vi "MultiGrid.vi"() -> ()   [LabVIEW 2014]
uses:
  <userlib>/Nanonis Prog Interface V5/Nanonis Prog Interface.lvlib
panel:
  in  "Cloud Grid":bool=TRUE
  in  "GridSettings":T1={"Imaging Current"=5e-11, "STS Current"=1e-09, "Start value (V)"=-0.05, "End value (V)"=0.05, "Number of points (0=no change)"=256, "File name"="single_mol_shortSTS", "DC pixel"=64.0, "Grid X"=0.0, "Grid Y"=0.0, "Sweeps"=8.0}
  in  "Polling (s)":u32=600
  out "Status":string="Waiting for grid to start"
  out "#Grids":i32=2
  out "MultiGrid":i32(listbox)
  # "0 for no change"
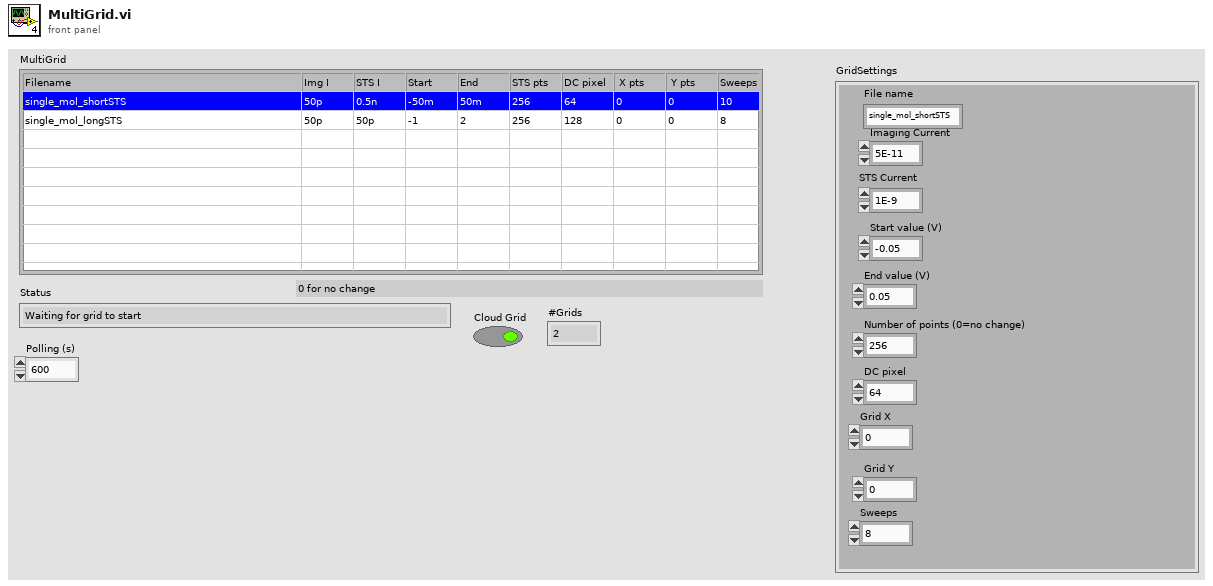
[diagram p1: front panel]
types:
  T1 = cluster{"Imaging Current":sgl, "STS Current":sgl, "Start value (V)":sgl, "End value (V)":sgl, "Number of points (0=no change)":i32, "File name":string, "DC pixel":dbl, "Grid X":dbl, "Grid Y":dbl, "Sweeps":dbl}
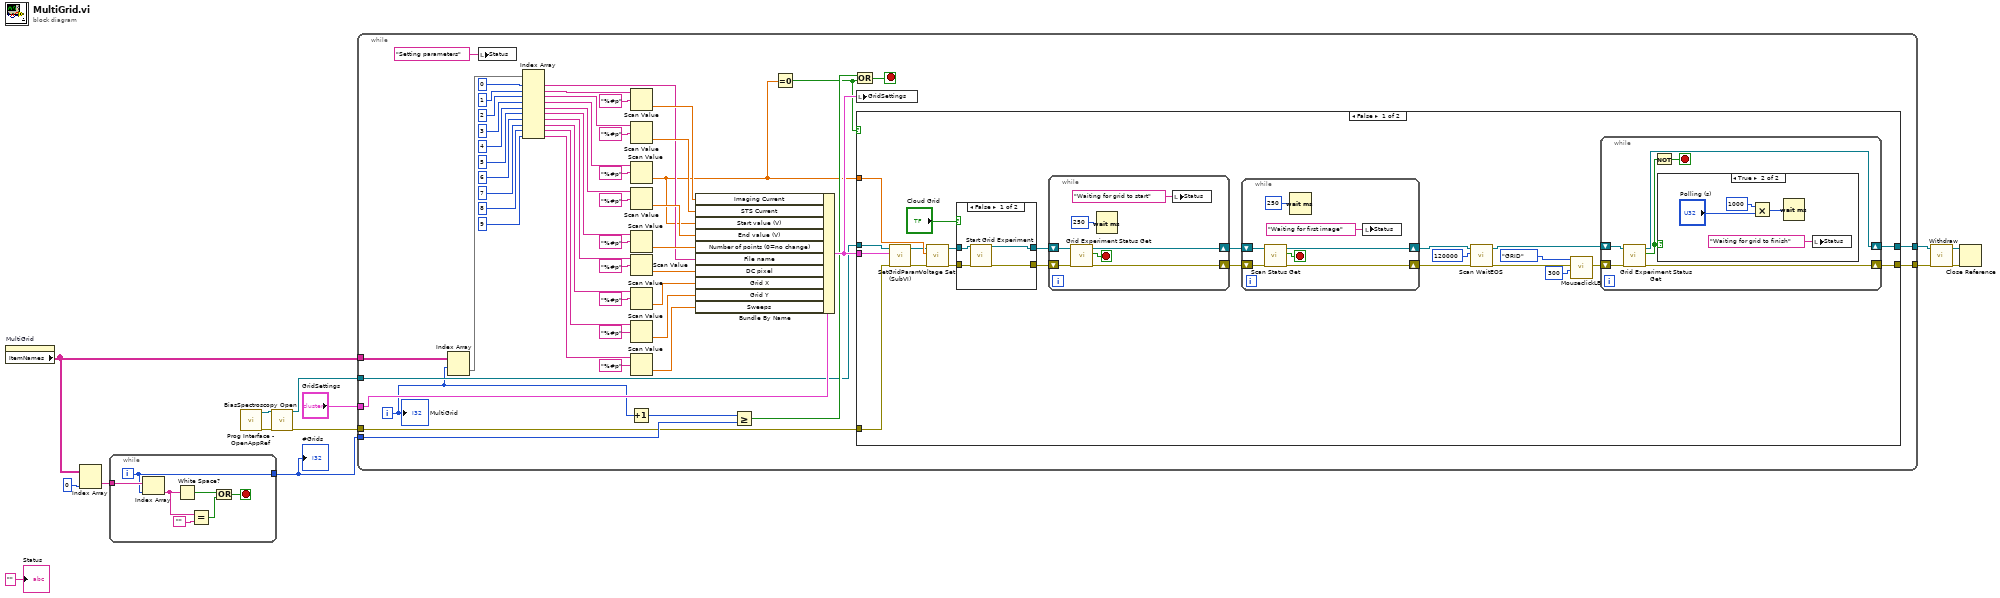
[diagram p0: block diagram]
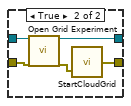
[diagram p2: hidden frame]
diagram:
  n1 = property on="MultiGrid" class="MCListbox (strict)"() -> ("ItemNames"=w12:string[][])  [unwired: 2 in, 2 out]
  n2 = Index Array(array=w12, index (col)=0 ("disabled index (col)")) -> (element=w10:string[])  [unwired: 1 in]
  n3 = while {
    tunnel: w10 -> [w21]
    tunnel: [w15] -> w7
    i -> [w15]
    stop <- w17 stop-if-true
    n4 = Index Array(array=w21, index=w15) -> (element=w20:string)
    n5 = White Space?(1:w20) -> (0:w18:bool)
    n6 = Equal?(x=w20, y="") -> (x = y?=w16:bool)
    n7 = Or(x=w18, y=w16) -> (x .or. y?=w17:bool)
  }
  "#Grids" <- w7
  n8 = call <userlib>:"Prog Interface - OpenAppRef.vi"() -> ("Error out"=w2:errorcluster, "Application reference"=w4:refnum<vi>)  [unwired: 6 in]
  n9 = call <userlib>:"BiasSpectroscopy Open.vi"("Application ref in"=w4, "Error in (no error)"=w2) -> ("Application ref out"=w3:refnum<vi>, "Error out"=w1:errorcluster)  [unwired: 12 in]
  n10 = while {
    tunnel: w12 -> [w74]
    tunnel: w3 -> [w29]
    tunnel: w1 -> [w28]
    tunnel: "GridSettings" -> [w68]
    tunnel: [w26] -> w14
    tunnel: [w30] -> w13
    tunnel: w7 -> [w31]
    i -> [w27]
    stop <- w25 stop-if-true
    n11 = Index Array(array=w74, index (row)=w27) -> (element=w66:string[])  [unwired: 1 in]
    n12 = local write "Status"("Setting parameters" ("Status")) -> ()
    n13 = Index Array(array=w66, index #1=0 ("index"), index #2=1 ("index"), index #3=2 ("index"), index #4=3 ("index"), index #5=4 ("index"), index #6=5 ("index"), index #7=6 ("index"), index #8=7 ("index"), index #9=8 ("index"), index #10=9 ("index")) -> (element #1=w38:string, element #2=w56:string, element #3=w54:string, element #4=w52:string, element #5=w51:string, element #6=w50:string, element #7=w49:string, element #8=w46:string, element #9=w45:string, element #10=w34:string)
    n14 = Increment(x=w27) -> (x+1=w24:i32)
    n15 = Scan Value(string=w56, format string="%#p") -> (value=w55:dbl)  [unwired: 1 in, 1 out]
    n16 = Scan Value(string=w54, format string="%#p") -> (value=w53:dbl)  [unwired: 1 in, 1 out]
    n17 = Scan Value(string=w52, format string="%#p") -> (value=w22:dbl)  [unwired: 1 in, 1 out]
    n18 = Scan Value(string=w51, format string="%#p") -> (value=w42:dbl)  [unwired: 1 in, 1 out]
    n19 = Scan Value(string=w50, format string="%#p") -> (value=w41:dbl)  [unwired: 1 in, 1 out]
    n20 = Scan Value(string=w49, format string="%#p") -> (value=w40:dbl)  [unwired: 1 in, 1 out]
    n21 = Scan Value(string=w46, format string="%#p") -> (value=w43:dbl)  [unwired: 1 in, 1 out]
    n22 = Scan Value(string=w45, format string="%#p") -> (value=w44:dbl)  [unwired: 1 in, 1 out]
    n23 = Scan Value(string=w34, format string="%#p") -> (value=w33:dbl)  [unwired: 1 in, 1 out]
    n24 = Bundle By Name(cluster=w68, "Imaging Current"=w55, "STS Current"=w53, "Start value (V)"=w22, "End value (V)"=w42, "Number of points (0=no change)"=w41, "File name"=w38, "DC pixel"=w40, "Grid X"=w43, "Grid Y"=w44, "Sweeps"=w33) -> (w39:T1)
    n25 = Greater Or Equal?(x=w24, y=w31) -> (x >= y?=w32:bool)
    n26 = Equal To 0?(x=w22) -> (x = 0?=w23:bool)
    n27 = Or(x=w32, y=w23) -> (x .or. y?=w25:bool)
    n28 = local write "GridSettings"(w39) -> ()
    n29 = case shown="False" w23 {
      tunnel: w39 -> [w97 _]
      tunnel: [w96 w131] -> w30
      tunnel: w29 -> [w95 w132]
      tunnel: w28 -> [w94 w131]
      tunnel: [w78 w132] -> w26
      tunnel: w22 -> [w77 _]
      frame False {
        n30 = call "SetGridParam (SubVI).vi"("error in (no error)"=w94, "GridSettings"=w97, "Application in"=w95) -> ("Error out"=w75:errorcluster, "Application ref out"=w76:refnum<vi>)  [unwired: 7 in]
        n31 = call <userlib>:"Voltage Set.vi"("Error in (no error)"=w75, "Bias (V)"=w77, "Application ref in"=w76) -> ("Error out"=w92:errorcluster, "Application ref out"=w93:refnum<vi>)  [unwired: 7 in]
        n32 = case shown="False" "Cloud Grid" {
          tunnel: w92 -> [w115 w118]
          tunnel: [w114 w119] -> w90
          tunnel: [w113 w117] -> w89
          tunnel: w93 -> [w112 w120]
          frame False {
            n33 = call <userlib>:"Start Grid Experiment.vi"("Application ref in"=w112, "error in (no error)"=w115) -> ("Application ref out"=w114:refnum<vi>, "error out"=w113:errorcluster)  [unwired: 16 in]
          }
          frame True {
            n34 = call <userlib>:"Open Grid Experiment.vi"("Application ref in"=w120, "error in (no error)"=w118) -> ("Application ref out"=w119:refnum<vi>, "error out"=w116:errorcluster)  [unwired: 16 in]
            n35 = call "StartCloudGrid.vi"("error in (no error)"=w116) -> ("error out"=w117:errorcluster)  [unwired: 1 in]
          }
        }
        n36 = while {
          shift-right: [w111] -> w83
          shift-left: w90 -> [w107]
          shift-right: [w106] -> w79
          shift-left: w89 -> [w110]
          stop <- w105 stop-if-true
          n37 = call <userlib>:"Grid Experiment Status Get.vi"("error in (no error)"=w110, "Application ref in"=w107) -> ("error out"=w106:errorcluster, "Running?"=w105:bool, "Application ref out"=w111:refnum<vi>)  [unwired: 7 in]
          n38 = Wait (ms)(milliseconds to wait=u32 250) -> ()  [unwired: 1 out]
          n39 = local write "Status"("Waiting for grid to start" ("Status")) -> ()
        }
        n40 = while {
          shift-right: [w102] -> w82
          shift-left: w83 -> [w103]
          shift-right: [w101] -> w81
          shift-left: w79 -> [w104]
          stop <- w100 stop-if-true
          n41 = call <userlib>:"Scan Status Get.vi"("error in (no error)"=w104, "Application ref in"=w103) -> ("error out"=w101:errorcluster, "Scanning?"=w100:bool, "Application ref out"=w102:refnum<vi>)  [unwired: 6 in]
          n42 = Wait (ms)(milliseconds to wait=u32 250) -> ()  [unwired: 1 out]
          n43 = local write "Status"("Waiting for first image" ("Status")) -> ()
        }
        n44 = call <userlib>:"Scan WaitEOS.vi"("error in (no error)"=w81, "Timeout in ms (-1)"=120000, "Application ref in"=w82) -> ("error out"=w85:errorcluster, "Application ref out"=w84:refnum<vi>)  [unwired: 4 in, 2 out]
        n45 = call "MouseclickLB.vi"("nMilliseconds"=300, "error in (no error)"=w85, "Click"=enum16{"Header", "TOPO", "STS", "GRID"}."GRID") -> ("error out"=w88:errorcluster)  [unwired: 8 in]
        n46 = while {
          shift-right: [w123] -> w78
          shift-left: w84 -> [w124]
          shift-right: [w121] -> w96
          shift-left: w88 -> [w122]
          stop <- w126 stop-if-true
          n47 = call <userlib>:"Grid Experiment Status Get.vi"("error in (no error)"=w122, "Application ref in"=w124) -> ("error out"=w121:errorcluster, "Running?"=w125:bool, "Application ref out"=w123:refnum<vi>)  [unwired: 7 in]
          n48 = Not(x=w125) -> (.not. x?=w126:bool)
          n49 = case shown="True" w125 {
            frame False {
            }
            frame True {
              n50 = Multiply(x=u32 1000, y="Polling (s)") -> (x*y=w129:u32)
              n51 = Wait (ms)(milliseconds to wait=w129) -> ()  [unwired: 1 out]
              n52 = local write "Status"("Waiting for grid to finish" ("Status")) -> ()
            }
          }
        }
      }
      frame True {
      }
    }
    "MultiGrid" <- w27
  }
  n53 = call <userlib>:"Withdraw.vi"("Error in (no error)"=w13, "Application ref in"=w14) -> ("Error out"=w5:errorcluster, "Application ref out"=w6:refnum<vi>)  [unwired: 8 in]
  n54 = Close Reference(reference=w6, error in (no error)=w5) -> ()  [unwired: 1 out]
  "Status" <- "" ("Status")
